vi "Is Bookmark.vi"(7 "Bookmark":T1, 8 "Error In":errorcluster, 11 "VI Bookmark":T2) -> (0 "Error Out":errorcluster, 3 "Is Bookmark":bool)   [LabVIEW 2017, in "Bookmark Manager.lvlib"]
uses:
  Bookmark Manager.lvlib
  VI Bookmark.ctl
  VI Information.ctl
  Application Information.ctl
  Eulogy/Public/Typedefs/Bookmarks.ctl
  Eulogy/Eulogy.lvlib
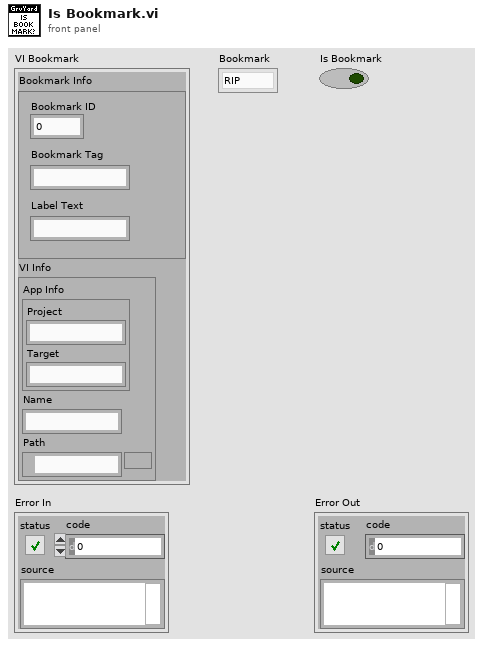
[diagram p1: front panel]
types:
  T1 = typedef "Eulogy.lvlib/Bookmarks.ctl" = enum16{"RIP", "Zombie"}
  T2 = typedef "Bookmark Manager.lvlib/VI Bookmark.ctl" = cluster{"Bookmark Info":cluster{"Bookmark ID":u32, "Bookmark Tag":string, "Label Text":string}, "VI Info":T3}
  T3 = typedef "Bookmark Manager.lvlib/VI Information.ctl" = cluster{"App Info":T4, "Name":string, "Path":path}
  T4 = typedef "Bookmark Manager.lvlib/Application Information.ctl" = cluster{"Project":string, "Target":string}
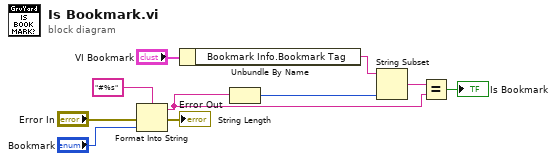
[diagram p0: block diagram]
diagram:
  n1 = Format Into String(format string="#%s", error in="Error In", "Bookmark") -> (resulting string=w3:string, error out=→"Error Out":errorcluster)  [unwired: 1 in]
  n2 = Unbundle By Name("VI Bookmark") -> ("Bookmark Info.Bookmark Tag"=w8:string)
  n3 = String Length(string=w3) -> (length=w10:i32)
  n4 = String Subset(string=w8, length (rest)=w10) -> (substring=w6:string)  [unwired: 1 in]
  n5 = Equal?(x=w6, y=w3) -> (x = y?=→"Is Bookmark":bool)
